vi "DLaserpowerAgilis.vi"(2 "error in (no error)":errorcluster) -> (0 "error out":errorcluster)   [LabVIEW 2011]
uses:
  <vilib>/Instr/_visa.llb/VISA Configure Serial Port (Instr).vi
  <vilib>/gmath/interp.llb/Interpolate 2D Scattered (1D).vi
  <vilib>/gmath/NI_AAL_Interpolation.lvlib
panel:
  out "VISA resource name":refnum<visa-resource-name>
  out "goto Motor pos":dbl
  out "Transmission":dbl
  in  "2D-Calibration (T,wl,out;)":string="0,600,68.15;0.01,600,65.28;0.05,600,61.69;0.12,600,58.02;0.25,600,53.15;0.75,600,38.15;0.89,600,32.83;0.975,600,27.7;1,600,23.2;0,1600,68.15;0.01,1600,65.28;0.05,1600,61.69;0.12,1600,58.02;0.25,1600,53.15;0.75,1600,38.15;0.89,1600,32.83;0.975,1600,27.7;1,1600,23.2;"
  out "Laser Wavelenth nm":dbl=751.0
  out "set IRPower in W":string
  # "This version is no regulator but controller:\ncalculate/estimate a single value and do it once\nIt has no feedback"
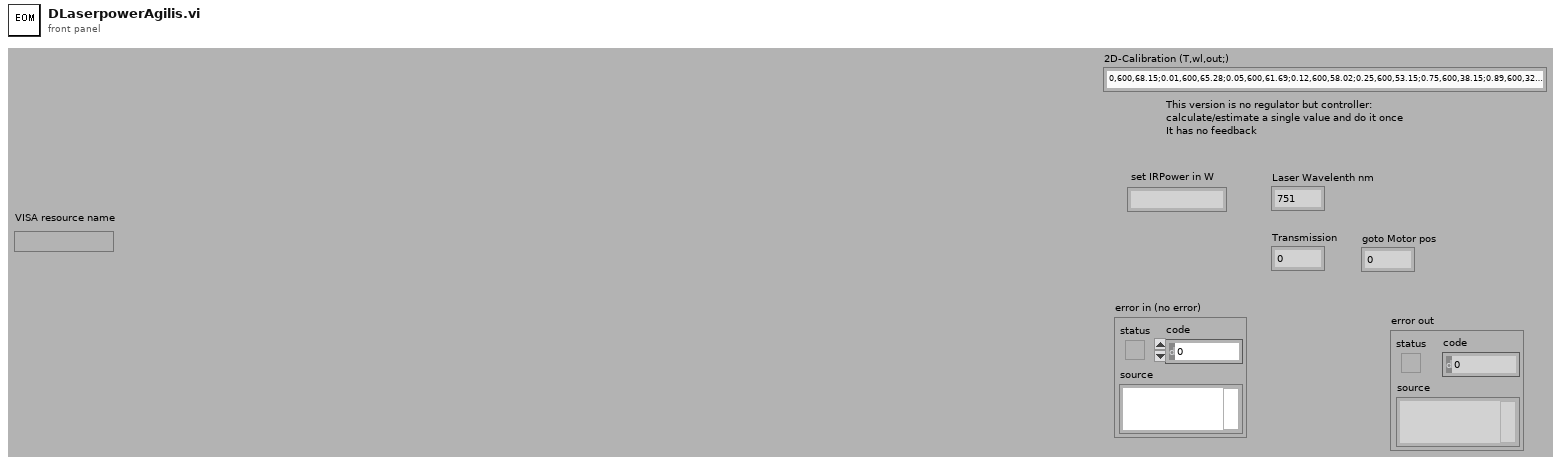
[diagram p1: front panel]
types:
  T1 = enum16{"None/#Datasets", "Clear", "TagValueOf#", "AddValues", "ReadValue", "ChangeValue", "Get all"}
  T2 = enum16{"NoOp", "GetStatus", "GetPosition", "SetPosition", "SetRelative", "GetError", "WriteRawAndRead", "clear", "switchOn"}
  T3 = cluster{"VISA resource name out":refnum<visa-resource-name>, "AxisID":i32}
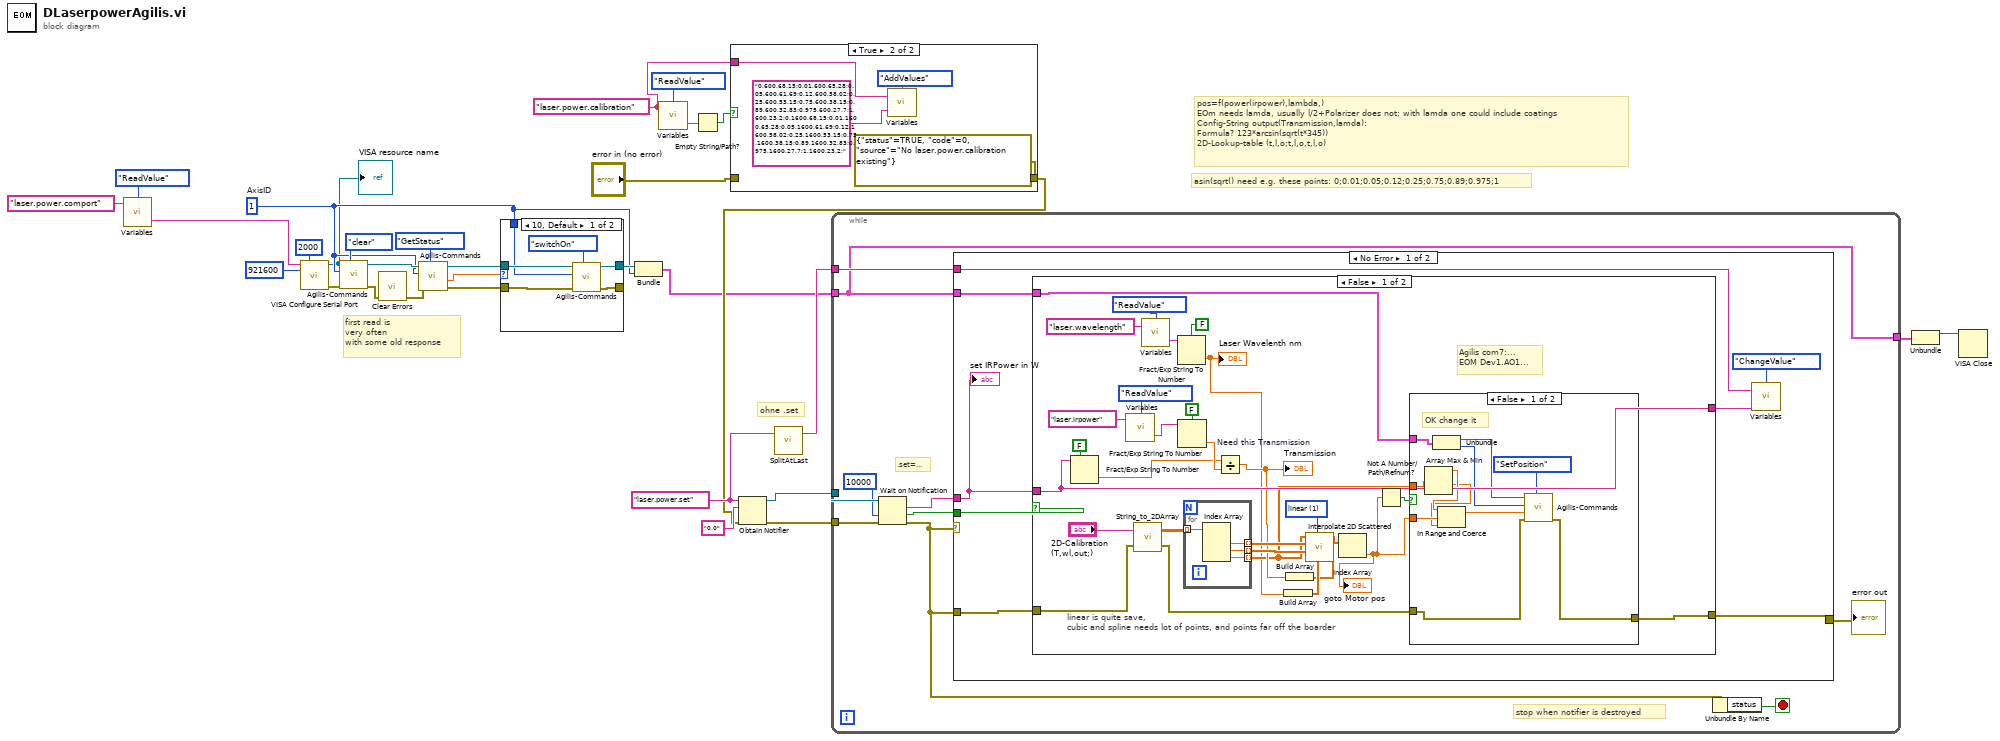
[diagram p0: block diagram]
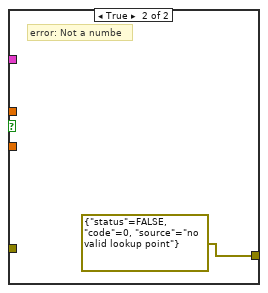
[diagram p4: hidden frame]
diagram:
  w7 = 1  # AxisID
  w23 = "laser.power.calibration" ("Tag in")
  w28 = "laser.power.set" ("name (unnamed)")
  # "first read is\nvery often \nwith some old response"
  # "asin(sqrt() need e.g. these points: 0;0.01;0.05;0.12;0.25;0.75;0.89;0.975;1"
  # "pos=f(power(irpower),lambda,)\nEOm needs lamda, usually l/2+Polarizer does not; with lamda one could include coatings \nConfig-String output(Transmission,lamda):\nFormula? 123*arcsin(sqrt(t*345))\n2D-Lookup-table (t,l,o;t,l,o,t,l,o)"
  # "ohne .set"
  n1 = call "Variables.vi"("Tag in"="laser.power.comport", "Command"=T1."ReadValue") -> ("value out"=w4:string)  [unwired: 1 in, 2 out]
  n2 = call-poly "VISA Configure Serial Port"("VISA resource name"=w4, "timeout (10sec)"=u32 2000, "baud rate (9600)"=u32 921600) -> ("VISA resource name out"=w3:refnum<visa-resource-name>, "error out"=w17:errorcluster)  [unwired: 11 in]
  "VISA resource name" <- w3
  n3 = call "Agilis-Commands.vi"("Command in"=T2."clear", "error in (no error)"=w17, "Axis in"=w7, "VISA Refnum in"=w3) -> ("error out"=w15:errorcluster, "VISA resource name out"=w16:refnum<visa-resource-name>)  [unwired: 4 in, 2 out]
  n4 = call <vilib>:"Clear Errors.vi"("error in (no error)"=w15) -> ("error out"=w14:errorcluster)  [unwired: 6 in]
  n5 = call "Agilis-Commands.vi"("Command in"=T2."GetStatus", "error in (no error)"=w14, "Axis in"=w7, "VISA Refnum in"=w16) -> ("error out"=w12:errorcluster, "value"=w13:dbl, "VISA resource name out"=w11:refnum<visa-resource-name>)  [unwired: 4 in, 1 out]
  n6 = case shown="10, Default" w13 {
    tunnel: w12 -> [w37 w39]
    tunnel: [w36 w39] -> _
    tunnel: w11 -> [w35 w38]
    tunnel: [w34 w38] -> w8
    tunnel: w7 -> [w32 _]
    frame 10, Default {
      n7 = call "Agilis-Commands.vi"("Command in"=T2."switchOn", "error in (no error)"=w37, "Axis in"=w32, "VISA Refnum in"=w35) -> ("error out"=w36:errorcluster, "VISA resource name out"=w34:refnum<visa-resource-name>)  [unwired: 4 in, 2 out]
    }
    frame 51 {
      # "OK"
    }
  }
  n8 = Bundle("VISA resource name out"=w8, "AxisID"=w7) -> (w20:T3)  [unwired: 1 in]
  n9 = call "Variables.vi"("Tag in"=w23, "Command"=T1."ReadValue") -> ("value out"=w25:string)  [unwired: 1 in, 2 out]
  n10 = Empty String/Path?(string/path=w25) -> (empty?=w24:bool)
  n11 = case shown="True" w24 {
    tunnel: w23 -> [_ w42]
    tunnel: "error in (no error)" -> [w40 _]
    tunnel: [w40 errorcluster {"status"=TRUE, "code"=0, "source"="No laser.power.calibration existing"} ("error in (no error)")] -> w21
    frame False {
      # "Calibration existing"
    }
    frame True {
      n12 = call "Variables.vi"("value"="0,600,68.15;0.01,600,65.28;0.05,600,61.69;0.12,600,58.02;0.25,600,53.15;0.75,600,38.15;0.89,600,32.83;0.975,600,27.7;1,600,23.2;0,1600,68.15;0.01,1600,65.28;0.05,1600,61.69;0.12,1600,58.02;0.25,1600,53.15;0.75,1600,38.15;0.89,1600,32.83;0.975,1600,27.7;1,1600,23.2;" ("2D-Calibration (T,wl,out;)"), "Tag in"=w42, "Command"=T1."AddValues") -> ()  [unwired: 3 out]
    }
  }
  n13 = Obtain Notifier(name (unnamed)=w28, notification data type="0.0", error in (no error)=w21) -> (notifier out=w30:refnum<notifier>, error out=w29:errorcluster)  [unwired: 1 in, 1 out]
  n14 = call "SplitAtLast.vi"("In-String"=w28) -> ("Front (default)"=w27:string)  [unwired: 1 in, 1 out]
  n15 = while {
    tunnel: w30 -> [w53]
    tunnel: w29 -> [w52]
    tunnel: w27 -> [w46]
    tunnel: w20 -> [w45]
    tunnel: [w45] -> w2
    stop <- w49 stop-if-true
    # "stop when notifier is destroyed"
    # ".set=..."
    n16 = Wait on Notification(notifier=w53, timeout in ms (-1)=10000, error in (no error)=w52) -> (notification=w51:string, timed out?=w48:bool, error out=w50:errorcluster)  [unwired: 2 out]
    n17 = case shown="No Error" w50 {
      tunnel: [w57 w110] -> w54
      tunnel: w50 -> [w58 w110]
      tunnel: w51 -> [w61 _]
      tunnel: w48 -> [w56 _]
      tunnel: w46 -> [w60 _]
      tunnel: w45 -> [w55 _]
      frame No Error {
        n18 = case shown="False" w56 {
          tunnel: w61 -> [w77 w109]
          tunnel: [w77 w109] -> w59
          tunnel: w58 -> [w74 w108]
          tunnel: [w69 w108] -> w57
          tunnel: w55 -> [w63 _]
          frame False {
            w82 = 1 items=["nearest", "linear", "cubic", "biharmonic spline "] ("method")
            # "Agilis com7:...\nEOM Dev1.AO1..."
            # "linear is quite save, \ncubic and spline needs lot of points, and points far off the boarder"
            n19 = Fract/Exp String To Number(use system decimal point (T)=FALSE, string=w77) -> (number=w78:dbl)  [unwired: 3 out]
            n20 = call "Variables.vi"("Tag in"="laser.irpower", "Command"=T1."ReadValue") -> ("value out"=w87:string)  [unwired: 1 in, 2 out]
            n21 = call "String_to_2DArray.vi"("error in (no error)"=w74, "String"="2D-Calibration (T,wl,out;)") -> ("error out"=w70:errorcluster, "Array"=w83:dbl[][])  [unwired: 2 in]
            n22 = call "Variables.vi"("Tag in"="laser.wavelength", "Command"=T1."ReadValue") -> ("value out"=w68:string)  [unwired: 1 in, 2 out]
            n23 = Fract/Exp String To Number(use system decimal point (T)=FALSE, string=w68) -> (number=w64:dbl)  [unwired: 3 out]
            "Laser Wavelenth nm" <- w64
            n24 = Fract/Exp String To Number(use system decimal point (T)=FALSE, string=w87) -> (number=w79:dbl)  [unwired: 3 out]
            n25 = for {
              tunnel: w83 -> [w107] mode=indexing
              tunnel: [w106] -> w86 mode=indexing
              tunnel: [w105] -> w85 mode=indexing
              tunnel: [w104] -> w72 mode=indexing
              n26 = Index Array(array=w107) -> (element #1=w106:dbl, element #2=w105:dbl, element #3=w104:dbl)  [unwired: 3 in]
            }
            n27 = Divide "Need this Transmission"(x=w78, y=w79) -> (x/y=w76:dbl)
            "Transmission" <- w76
            n28 = Build Array(w64) -> (w81:dbl[])
            n29 = Build Array(w76) -> (w75:dbl[])
            n30 = call-poly <vilib>:"Interpolate 2D Scattered.vi"("Yi"=w81, "method"=w82, "Xi"=w75, "Y"=w85, "X"=w86, "Z"=w72) -> ("Zi"=w80:dbl[])  [unwired: 4 in, 1 out]
            n31 = Index Array(array=w80) -> (element=w71:dbl)  [unwired: 1 in]
            "goto Motor pos" <- w71
            n32 = Not A Number/Path/Refnum?(number/path/refnum=w71) -> (NaN/Path/Refnum?=w73:bool)
            n33 = case shown="False" w73 {
              tunnel: w72 -> [w102 _]
              tunnel: w71 -> [w101 _]
              tunnel: w70 -> [w93 _]
              tunnel: [w92 errorcluster {"status"=FALSE, "code"=0, "source"="no valid lookup point"} ("error out")] -> w69
              tunnel: w63 -> [w96 _]
              frame False {
                # "OK change it"
                n34 = Array Max & Min(array=w102) -> (max value=w100:dbl, min value=w99:dbl)  [unwired: 2 out]
                n35 = Unbundle(w96) -> ("VISA resource name out"=w95:refnum<visa-resource-name>, "AxisID"=w94:i32)
                n36 = In Range and Coerce(upper limit=w100, x=w101, lower limit=w99) -> (coerced(x)=w97:dbl)  [unwired: 1 out]
                n37 = call "Agilis-Commands.vi"("Command in"=T2."SetPosition", "error in (no error)"=w93, "Value"=w97, "Axis in"=w94, "VISA Refnum in"=w95) -> ("error out"=w92:errorcluster)  [unwired: 3 in, 3 out]
              }
              frame True {
                # "error: Not a numbe"
              }
            }
          }
          frame True {
            # "timeout \ncould check power, status ..."
          }
        }
        n38 = call "Variables.vi"("value"=w59, "Tag in"=w60, "Command"=T1."ChangeValue") -> ()  [unwired: 3 out]
        "set IRPower in W" <- w61
      }
      frame Error {
      }
    }
    "error out" <- w54
    n39 = Unbundle By Name(w50) -> ("status"=w49:bool)
  }
  n40 = Unbundle(w2) -> ("VISA resource name out"=w1:refnum<visa-resource-name>)  [unwired: 1 out]
  n41 = VISA Close(VISA resource name=w1) -> ()  [unwired: 1 in, 1 out]
